vi "Get Watlow Data.vi"(8 "Error IN":errorcluster) -> (0 "Error OUT":errorcluster, 2 "Setpoint Changed":bool, 3 "Tank Temp Variables":T1)   [LabVIEW 2013]
uses:
  Controls/Tank Temp Variables.ctl
  Watlow Modbus/Modbus Mode.ctl
  Watlow Modbus/Modbus Variable.ctl
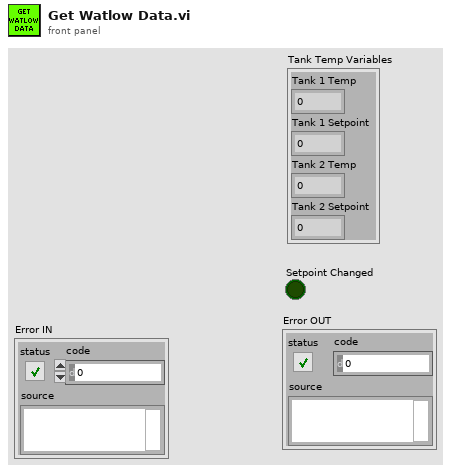
[diagram p1: front panel]
types:
  T1 = typedef "Tank Temp Variables.ctl" = cluster{"Tank 1 Temp":sgl, "Tank 1 Setpoint":sgl, "Tank 2 Temp":sgl, "Tank 2 Setpoint":sgl}
  T2 = typedef "Modbus Variable.ctl" = enum16{"Temperature", "Setpoint"}
  T3 = typedef "Modbus Mode.ctl" = enum16{"Init", "Tank 1 Write", "Tank 2 Write", "Tank 1 Read", "Tank 2 Read"}
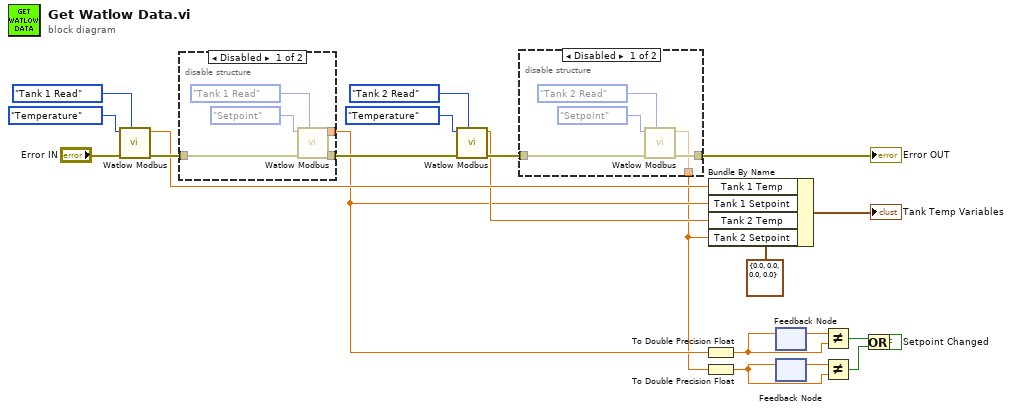
[diagram p0: block diagram]
diagram:
  n1 = call "Watlow Modbus.vi"("Modbus Mode"=Modbus_Mode."Tank 1 Read", "Error IN"="Error IN", "Variable"=Modbus_Variable."Temperature") -> ("Error OUT"=w18:errorcluster, "Data Read"=w13:sgl)  [unwired: 7 in]
  n2 = disable-structure shown="Disabled" {
    disable-tunnel: w18 -> [w25 _]
    disable-tunnel: [w24 _] -> w17
    disable-tunnel: [w23 _] -> w3
    frame Disabled {
      n3 = call "Watlow Modbus.vi"("Modbus Mode"=Modbus_Mode."Tank 1 Read", "Error IN"=w25, "Variable"=Modbus_Variable."Setpoint") -> ("Error OUT"=w24:errorcluster, "Data Read"=w23:sgl)  [unwired: 7 in]
    }
    frame Enabled {
    }
  }
  n4 = call "Watlow Modbus.vi"("Modbus Mode"=Modbus_Mode."Tank 2 Read", "Error IN"=w17, "Variable"=Modbus_Variable."Temperature") -> ("Error OUT"=w16:errorcluster, "Data Read"=w12:sgl)  [unwired: 7 in]
  n5 = disable-structure shown="Disabled" {
    disable-tunnel: w16 -> [w30 _]
    disable-tunnel: [w29 _] -> w14
    disable-tunnel: [w28 _] -> w2
    frame Disabled {
      n6 = call "Watlow Modbus.vi"("Modbus Mode"=Modbus_Mode."Tank 2 Read", "Error IN"=w30, "Variable"=Modbus_Variable."Setpoint") -> ("Error OUT"=w29:errorcluster, "Data Read"=w28:sgl)  [unwired: 7 in]
    }
    frame Enabled {
    }
  }
  "Error OUT" <- w14
  n7 = To Double Precision Float(number=w3) -> (double precision float=w8:dbl)
  n8 = To Double Precision Float(number=w2) -> (double precision float=w6:dbl)
  n9 = Bundle By Name(cluster=T1 {"Tank 1 Temp"=0.0, "Tank 1 Setpoint"=0.0, "Tank 2 Temp"=0.0, "Tank 2 Setpoint"=0.0} ("output cluster"), "Tank 1 Temp"=w13, "Tank 1 Setpoint"=w3, "Tank 2 Temp"=w12, "Tank 2 Setpoint"=w2) -> (→"Tank Temp Variables":T1)
  n10 = feedback #1() -> (w9:dbl)  [unwired: 1 in]
  n11 = feedback-in #1(w8) -> ()
  n12 = feedback #2() -> (w7:dbl)  [unwired: 1 in]
  n13 = feedback-in #2(w6) -> ()
  n14 = Not Equal?(x=w9, y=w8) -> (x != y?=w5:bool)
  n15 = Not Equal?(x=w7, y=w6) -> (x != y?=w4:bool)
  n16 = Or(x=w5, y=w4) -> (x .or. y?=→"Setpoint Changed":bool)
